vi "Update Account Balance.vi"(8 "error in (no error)":errorcluster, 10 "Account PIN":string, 11 "New Amount":dbl) -> (0 "error out":errorcluster)   [LabVIEW 2025]
doc: "Update the account balance in the csv file with the new account balance."
uses:
  <vilib>/Utility/file.llb/Read Delimited Spreadsheet (string).vi
  <vilib>/Utility/file.llb/Write Delimited Spreadsheet (string).vi
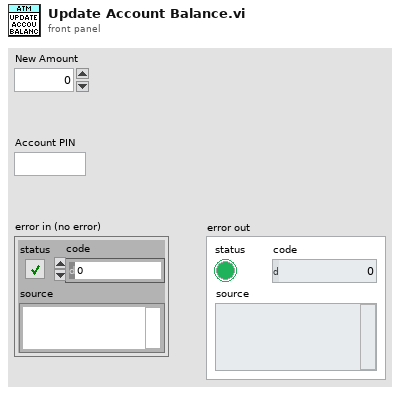
[diagram p1: front panel]
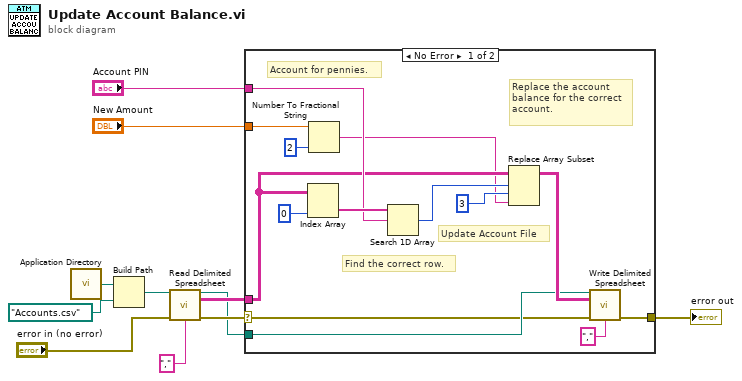
[diagram p0: block diagram]
diagram:
  n1 = call <vilib>:"Application Directory.vi"() -> ("Application Directory"=w11:path)
  n2 = Build Path(base path=w11, name or relative path=path "Accounts.csv") -> (appended path=w9:path)
  n3 = call-poly <vilib>:"Read Delimited Spreadsheet.vi"("file path (dialog if empty)"=w9, "error in (no error)"="error in (no error)", "delimiter (\\t)"="," ("delimiter (\\t)")) -> ("new file path (Not A Path if cancelled)"=w1:path, "all rows"=w5:string[][], "error out"=w7:errorcluster)  [unwired: 7 in, 3 out]
  n4 = case shown="No Error" w7 {
    selector: w7 -> [w14 w26]
    tunnel: w5 -> [w22 _]
    tunnel: [w13 w26] -> w4
    tunnel: "Account PIN" -> [w23 _]
    tunnel: "New Amount" -> [w19 _]
    tunnel: w1 -> [w15 _]
    frame No Error {
      # "Update Account File"
      # "Account for pennies."
      # "Replace the account \nbalance for the correct\naccount."
      # "Find the correct row."
      n5 = Index Array(array=w22, index (col)=0) -> (element=w24:string[])  [unwired: 1 in]
      n6 = Number To Fractional String(number=w19, precision (6)=i16 2) -> (F-format string=w17:string)  [unwired: 2 in]
      n7 = Search 1D Array(1D array=w24, element=w23) -> (index of element=w21:i32)  [unwired: 1 in]
      n8 = Replace Array Subset(array=w22, new element=w17, index (row)=w21, index (col)=3) -> (w16:string[][])
      n9 = call-poly <vilib>:"Write Delimited Spreadsheet.vi"("file path (dialog if empty)"=w15, "2D data"=w16, "error in (no error)"=w14, "delimiter (\\t)"="," ("delimiter (\\t)")) -> ("error out"=w13:errorcluster)  [unwired: 10 in, 1 out]
    }
    frame Error {
    }
  }
  "error out" <- w4
